vi "配置串口.vi"(5 "Parity":i32(ring) items=["None", "Odd", "Even", "Mark", "Space"], 6 "Stop Bits":i32(ring)=1 items=["None", "One", "Two", "OnePointFive"], 7 "Data Bits":i32=8, 8 "error in (no error)":errorcluster caption="错误输入（无错误）", 9 "Baud Rate":i32=9600, 10 "Port Name":string="COM1", 11 "COM 输入":refnum<class "串口.lvclass"> caption="DNL_LabVIEW Object in") -> (0 "error out":errorcluster caption="错误输出", 3 "COM 输出":refnum<class "串口.lvclass"> caption="DNL_LabVIEW Object out")   [LabVIEW 2012, in "串口.lvclass"]
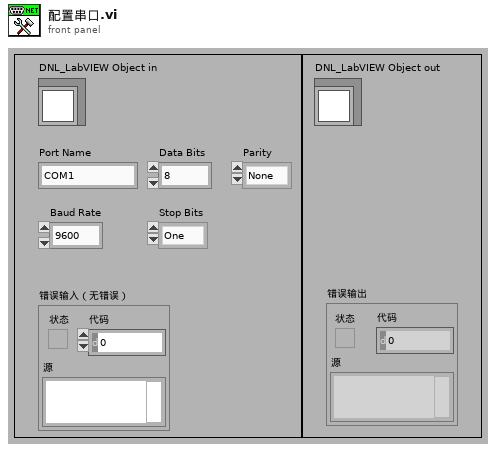
[diagram p1: front panel]
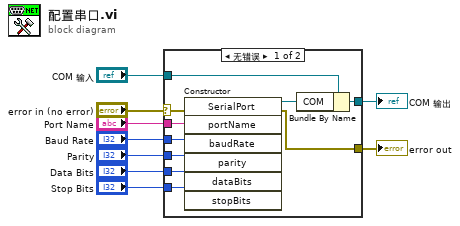
[diagram p0: block diagram]
diagram:
  n1 = case shown="无错误" "error in (no error)" {
    selector: "error in (no error)" -> [w19 w21]
    tunnel: [w10 w21] -> w8
    tunnel: [w11 w20] -> w6
    tunnel: "COM 输入" -> [w12 w20]
    tunnel: "Port Name" -> [w18 _]
    tunnel: "Baud Rate" -> [w17 _]
    tunnel: "Parity" -> [w16 _]
    tunnel: "Data Bits" -> [w15 _]
    tunnel: "Stop Bits" -> [w14 _]
    frame No Error {
      n2 = constructor class="SerialPort"(error in=w19, "portName"=w18, "baudRate"=w17, "parity"=w16, "dataBits"=w15, "stopBits"=w14) -> (reference out=w13:refnum<k24>, error out=w10:errorcluster)  [unwired: 2 in, 6 out]
      n3 = Bundle By Name(cluster=w12, "COM"=w13) -> (w11:refnum<class "串口.lvclass">)
    }
    frame Error {
    }
  }
  "error out" <- w8
  "COM 输出" <- w6
